vi "Set Firmware Version.vi"(11 "Tool Firmware Version String":string) -> ()   [LabVIEW 2015, in "Tool Cfg.lvlib"]
uses:
  Tool Cfg.lvlib
  ConfigGLOB.vi
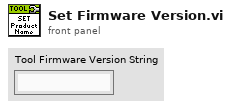
[diagram p1: front panel]
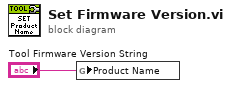
[diagram p0: block diagram]
diagram:
  n1 = global write "ConfigGLOB.vi" "Product Name"("Tool Firmware Version String") -> ()
